vi "EventLog.Init.vi"(8 "error in":errorcluster) -> (0 "error out":errorcluster)   [LabVIEW 2016]
uses:
  EventLog.Buffer.Action.ctl
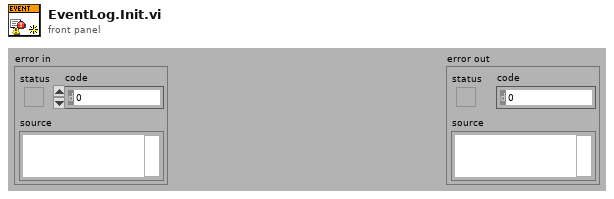
[diagram p1: front panel]
types:
  T1 = typedef "EventLog.Buffer.Action.ctl" = enum16{"init", "re-init", "clear", "set translator", "add", "get", "get unsaved"}
  T2 = enum32{"Bad", "Idle", "Run top level", "Running"}
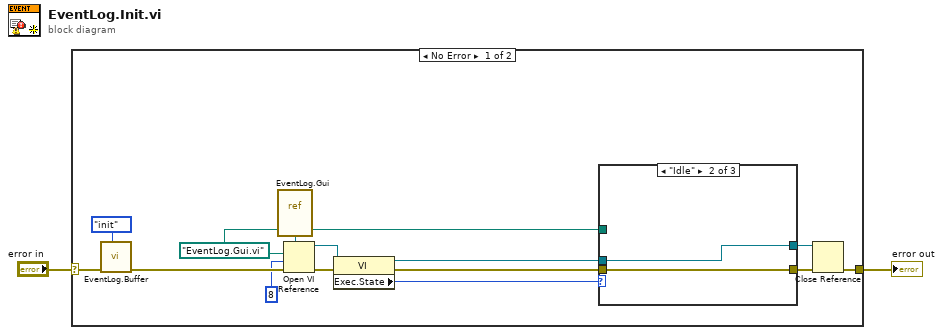
[diagram p0: block diagram]
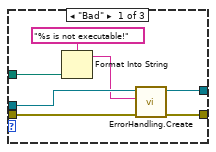
[diagram p2: hidden frame]
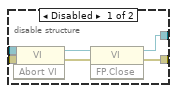
[diagram p4: hidden frame]
diagram:
  n1 = case shown="No Error" "error in" {
    selector: "error in" -> [w11 w37]
    tunnel: [w6 w37] -> w2
    frame No Error {
      w3 = path "EventLog.Gui.vi" ("vi path")
      n2 = call "EventLog.Buffer.vi"("action (get)"=EventLog.Buffer.Action."init" ("action (read)"), "error in"=w11) -> ("error out"=w10:errorcluster)  [unwired: 6 in, 3 out]
      n3 = vi-ref "EventLog.Gui.vi"() -> (w13:refnum<vi>)
      n4 = Open VI Reference(type specifier VI Refnum (for type only)=w13, vi path=w3, options=8, error in (no error)=w10) -> (vi reference=w15:refnum<vi>, error out=w16:errorcluster)  [unwired: 2 in]
      n5 = property class="VI"(reference=w15, error in=w16) -> (reference out=w8:refnum<vi>, error out=w9:errorcluster, "Exec.State"=w14:T2)
      n6 = case shown="\"Idle\"" w14 {
        tunnel: [w20 w24 w25] -> w7
        tunnel: w9 -> [w21 w24 w28]
        tunnel: w8 -> [w22 w23 w27]
        tunnel: [w22 w23 w26] -> w5
        tunnel: w3 -> [w19 _ _]
        frame "Bad" {
          n7 = Format Into String(format string="%s is not executable!" ("explanation"), w19) -> (resulting string=w17:string)  [unwired: 2 in, 1 out]
          n8 = call "ErrorHandling.Create.vi"("error in"=w21, "explanation"=w17) -> ("error out"=w20:errorcluster)  [unwired: 9 in]
        }
        frame "Idle" {
        }
        frame "Run top level", "Running" {
          n9 = disable-structure shown="Enabled" {
            disable-tunnel: w28 -> [w34 w36]
            disable-tunnel: w27 -> [w33 w35]
            disable-tunnel: [w30 w35] -> w26
            disable-tunnel: [w29 w36] -> w25
            frame Disabled {
              n10 = invoke class="VI" method="Abort VI"(reference=w33, error in=w34) -> (reference out=w31:refnum<vi>, error out=w32:errorcluster)  [unwired: 1 in, 1 out]
              n11 = invoke class="VI" method="FP.Close"(reference=w31, error in=w32) -> (reference out=w30:refnum<vi>, error out=w29:errorcluster)  [unwired: 1 in, 1 out]
            }
            frame Enabled {
            }
          }
        }
      }
      n12 = Close Reference(reference=w5, error in (no error)=w7) -> (error out=w6:errorcluster)
    }
    frame Error {
    }
  }
  "error out" <- w2
